vi "transRec.vi"() -> ()   [LabVIEW 2015]
uses:
  <vilib>/imath/engines/lvmath/Functions/Error Handling/error.ctl
  <instrlib>/niUSRP/niUSRP Write Tx Data (2D CDB).vi
  <instrlib>/niUSRP/niUSRP Fetch Rx Data (CDB WDT).vi
  <vilib>/measure/maspectr.llb/FFT Power Spectrum for 1 Chan (CDB).vi
  <vilib>/imath/engines/lvmath2/RunTimeEngine/Managers/WorkSpace/UID Generator.vi
  <vilib>/imath/engines/lvmath2/RunTimeEngine/NonStaticBuiltInFunctions/Manual/NIMS_NS_load.vi
  <vilib>/imath/engines/lvmath/Plug In/Control Design/NonStaticBuiltInFunctions/NIMS_NS_repeatmx.vi
  <vilib>/imath/engines/lvmath2/RunTimeEngine/RunTimeType/NIMS_RunTimeType_From StrictType (excl LVString).vi
  <instcachedir>/0/NIMS_RunTimeType_From StrictType (excl LVString)_EB1C38A9BC5048DA9ABDA8F781E54D21.lvgen/NIMS_RunTimeType_From StrictType (excl LVString)_EB1C38A9BC5048DA9ABDA8F781E54D21_000.vi
  <vilib>/imath/engines/lvmath2/RunTimeEngine/Managers/SymbolTable/Write Variable.vi
  <vilib>/imath/engines/lvmath/Plug In/Control Design/RunTimeSymbolToken/NIMS_CD_RunTimeSymbolToken_ResolveSymbol.vi
  <instcachedir>/0/NIMS_CD_RunTimeSymbolToken_ResolveSymbol_2FAE1C21E82D46CA9B9EE006FDCE72DC.lvgen/NIMS_CD_RunTimeSymbolToken_ResolveSymbol_2FAE1C21E82D46CA9B9EE006FDCE72DC_000.vi
  <vilib>/imath/engines/lvmath2/RunTimeEngine/LocalVariableDefStatement/MC_LocalVariableDefStatement_Display.vi
  <vilib>/imath/engines/lvmath2/RunTimeEngine/RunTimeSymbolToken/NIMS_RunTimeSymbolToken_ReadVariable-1out.vi
  <instcachedir>/0/NIMS_CD_RunTimeSymbolToken_ResolveSymbol_2FAE1C21E82D46CA9B9EE006FDCE72DC.lvgen/NIMS_CD_RunTimeSymbolToken_ResolveSymbol_2FAE1C21E82D46CA9B9EE006FDCE72DC_001.vi
  <vilib>/imath/engines/lvmath/Functions/Error Handling/MergeErrorsWrapper.vi
  <vilib>/imath/engines/lvmath2/RunTimeEngine/ArithmeticOperatorToken/NIMS_NS_ArithmeticOperator_rightdiv.vi
  <vilib>/imath/engines/lvmath/Plug In/Control Design/ArithmeticOperatorToken/NIMS_CD_NS_ArithmeticOperator_multmx.vi
  <vilib>/imath/engines/lvmath2/RunTimeEngine/CommandStatement/NIMS_CommandStatement_MaskErr.vi
  <vilib>/imath/engines/lvmath2/RunTimeEngine/Managers/SymbolTable/Read Variable.vi
  <vilib>/imath/engines/lvmath2/RunTimeEngine/RunTimeType/NIMS_RunTimeType_Get Case Value.vi
  <vilib>/imathl/engines/lvmath/Functions/Error Handling/Create Error.vi
  <vilib>/imath/engines/lvmath2/RunTimeEngine/RunTimeType/NIMS_RunTimeType_To Numeric.vi
  <instcachedir>/0/NIMS_RunTimeType_To Numeric_B134FEC7BFC54ED5998F4CFD2EE98288.lvgen/NIMS_RunTimeType_To Numeric_B134FEC7BFC54ED5998F4CFD2EE98288_000.vi
  <vilib>/imath/engines/lvmath/Plug In/_Char/RunTimeType/NIMS_CH_RunTimeType_To Character 2D.vi
  <vilib>/imath/engines/lvmath/Plug In/_Char/NIMS_CH_Character 2D to U8 2D.vi
  <vilib>/imath/engines/lvmath2/RunTimeEngine/NodeEndStatement/MC_NodeEndStatement_Dispose.vi
  <vilib>/imath/engines/lvmath2/RunTimeEngine/NodeEndStatement/NIMS_NodeEndStatement_Output.vi
  <instcachedir>/0/NIMS_NodeEndStatement_Output_53EC0D466D134D7ABD903AC30B43404B.lvgen/NIMS_NodeEndStatement_Output_53EC0D466D134D7ABD903AC30B43404B_003.vi
  <vilib>/imath/engines/lvmath2/RunTimeEngine/ErrorHandling/NIMS_Finalize Error.vi
  <vilib>/imath/engines/lvmath2/RunTimeEngine/Managers/SymbolTable/NIMS_WorkSpace.lvlib
  <vilib>/measure/NI_MAPro.lvlib
panel:
  out "Baseband Power Spectrum":cluster{"f0":dbl, "df":dbl, "magnitude":dbl[]}(graph)
  out "Waveform Graph 2":dbl[][](graph)
  out "Waveform Graph":dbl[][](graph)
  in  "error in rx":errorcluster
  in  "device names rx":refnum<k15>
  in  "active antenna x2":string
  in  "active antenna x1":string
  out "coerced gain x2":dbl format="%#_6f"
  out "coerced carrier frequency x2":dbl=100000.0 format="%#_6p"
  out "coerced IQ rate x2":dbl=100000.0 format="%#_6p"
  in  "gain x2":dbl format="%#_6f"
  in  "IQ rate x2":dbl=100000.0 format="%#_6p"
  in  "carrier frequency x2":dbl=100000.0 format="%#_6p"
  in  "device names x2":refnum<k15>
  in  "error in 2":errorcluster
  in  "stop button x2":bool
  in  "number of samples":i64=100000
  in  "stop button rx":bool
  in  "active antenna rx":string
  out "coerced carrier frequency rx":dbl=100000.0 format="%#_6p"
  out "coerced gain rx":dbl format="%#_6f"
  out "coerced IQ rate rx":dbl=100000.0 format="%#_6p"
  in  "gain rx":dbl format="%#_6f"
  in  "carrier frequency rx":dbl=100000.0 format="%#_6p"
  in  "IQ rate rx":dbl=100000.0 format="%#_6p"
  in  "stop button x1":bool
  out "coerced gain x1":dbl format="%#_6f"
  out "coerced carrier frequency x1":dbl=100000.0 format="%#_6p"
  out "coerced IQ rate x1":dbl=100000.0 format="%#_6p"
  in  "gain x1":dbl format="%#_6f"
  in  "IQ rate x1":dbl=100000.0 format="%#_6p"
  in  "carrier frequency x1":dbl=100000.0 format="%#_6p"
  in  "device names x1":refnum<k15>
  in  "error in 1":errorcluster
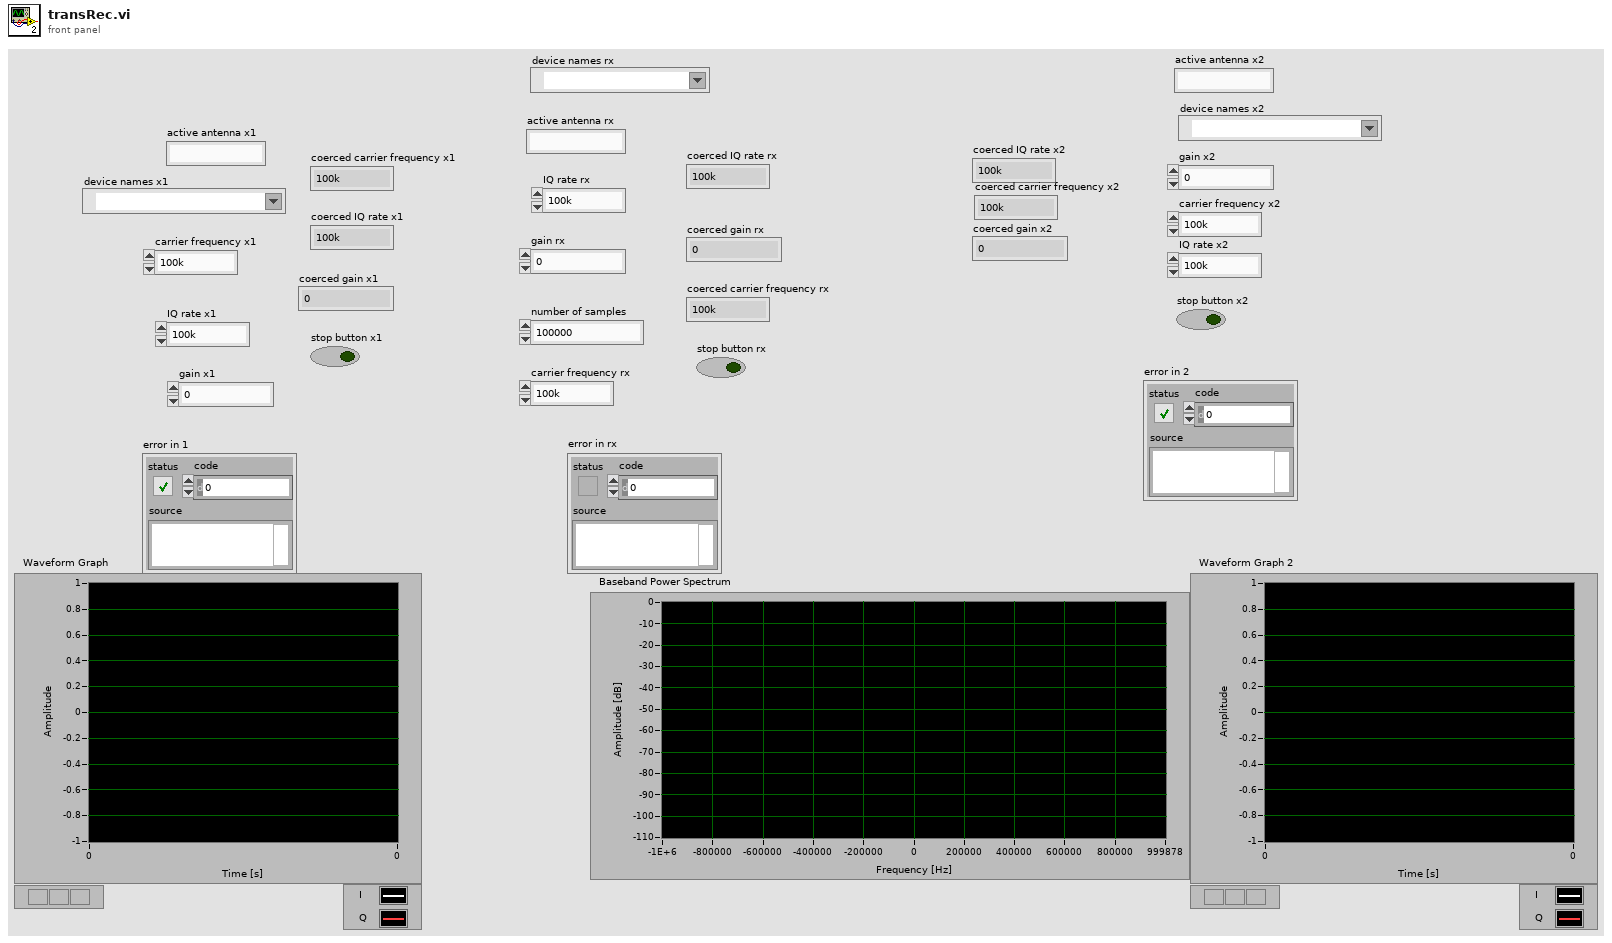
[diagram p1: front panel]
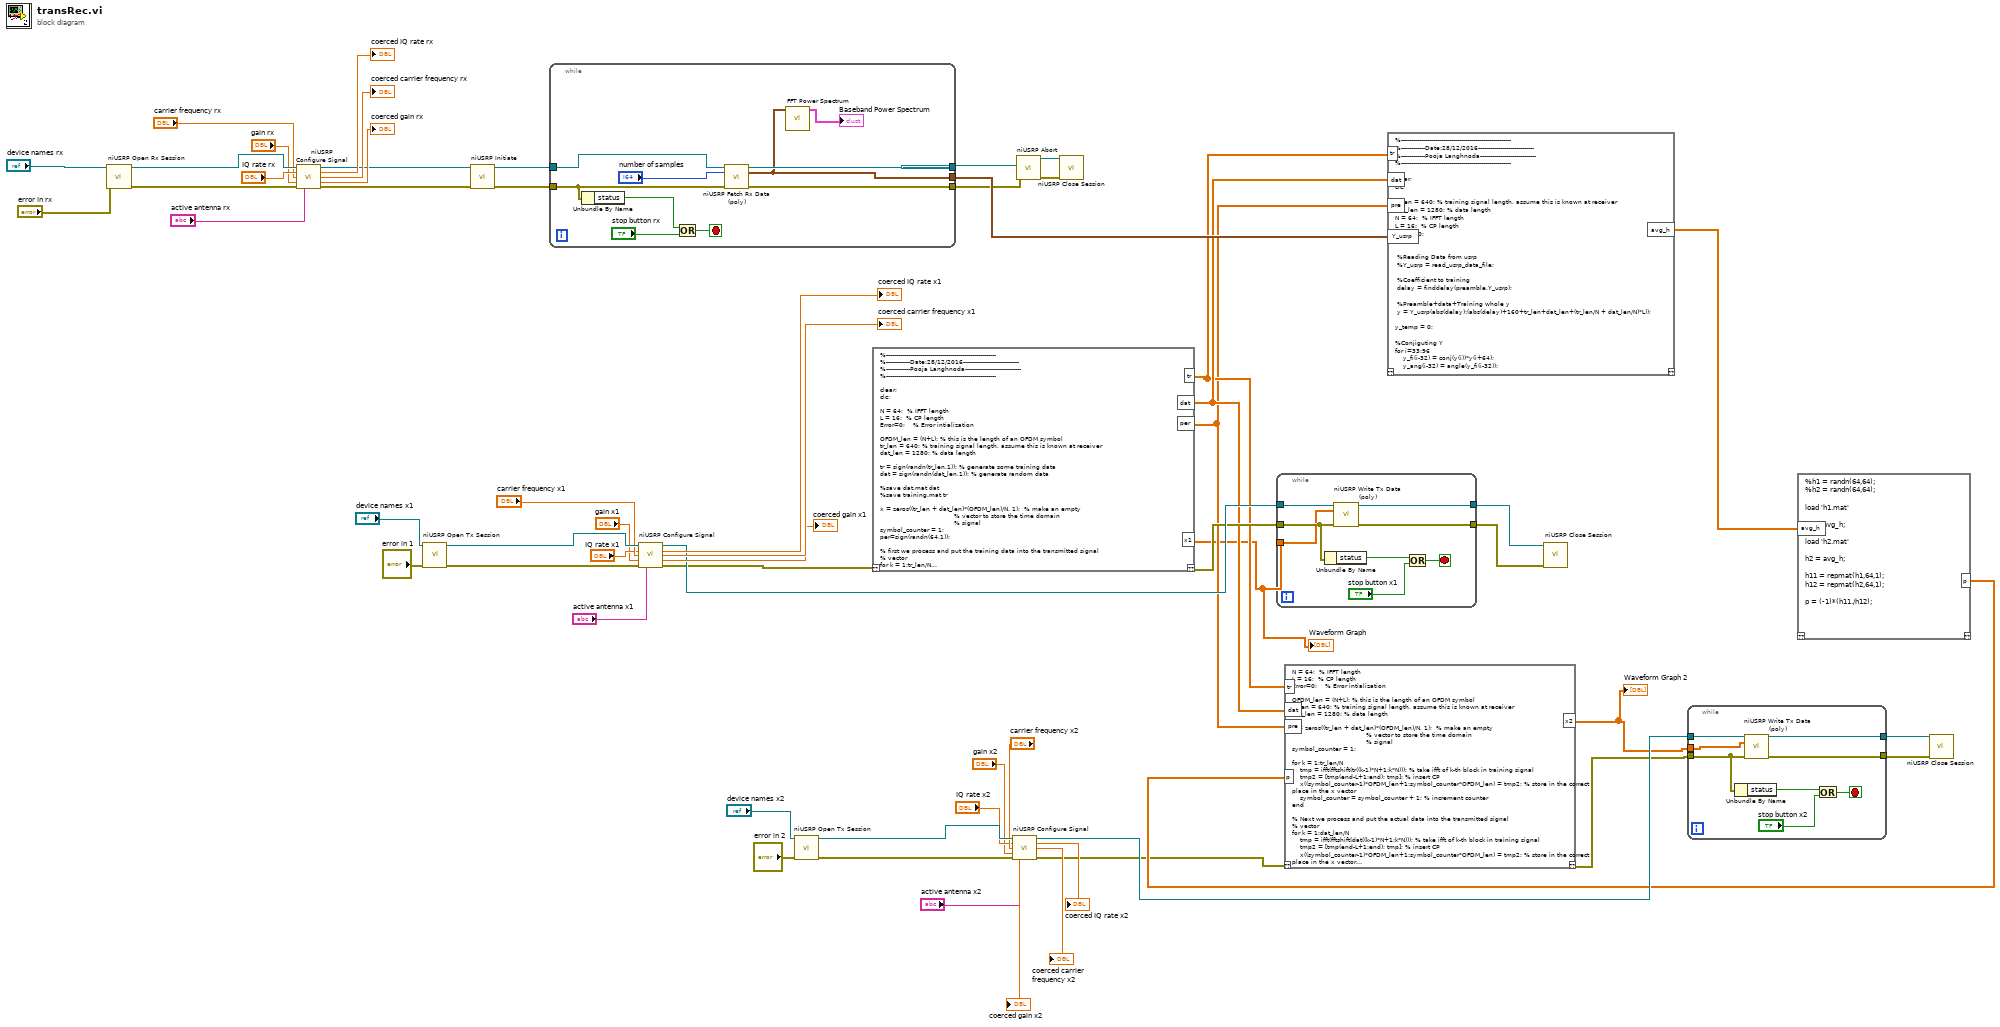
[diagram p0: block diagram]
diagram:
  n1 = call <instrlib>:"niUSRP Open Rx Session.vi"("device names"="device names rx", "error in (no error)"="error in rx") -> ("session handle out"=w45:refnum<k15>, "error out"=w44:errorcluster)  [unwired: 12 in]
  n2 = call <instrlib>:"niUSRP Configure Signal.vi"("session handle"=w45, "IQ rate"="IQ rate rx", "carrier frequency"="carrier frequency rx", "gain"="gain rx", "error in (no error)"=w44, "active antenna"="active antenna rx") -> ("session handle out"=w38:refnum<k15>, "coerced IQ rate"=→"coerced IQ rate rx":dbl, "coerced carrier frequency"=→"coerced carrier frequency rx":dbl, "coerced gain"=→"coerced gain rx":dbl, "error out"=w37:errorcluster)  [unwired: 5 in]
  n3 = call <instrlib>:"niUSRP Open Tx Session.vi"("device names"="device names x1", "error in (no error)"="error in 1") -> ("session handle out"=w58:refnum<k15>, "error out"=w50:errorcluster)  [unwired: 12 in]
  n4 = call <instrlib>:"niUSRP Initiate.vi"("session handle"=w38, "error in (no error)"=w37) -> ("session handle out"=w35:refnum<k15>, "error out"=w34:errorcluster)  [unwired: 12 in]
  n5 = while {
    tunnel: w35 -> [w65]
    tunnel: [w66] -> w30
    tunnel: w34 -> [w62]
    tunnel: [w61] -> w33
    tunnel: [w63] -> w29
    stop <- w67 stop-if-true
    n6 = Unbundle By Name(w62) -> ("status"=w68:bool)
    n7 = Or(x=w68, y="stop button rx") -> (x .or. y?=w67:bool)
    n8 = call-poly <instrlib>:"niUSRP Fetch Rx Data (poly).vi"("session handle"=w65, "number of samples"="number of samples", "error in (no error)"=w62) -> ("session handle out"=w66:refnum<k15>, "data"=w61:waveform(cdb), "error out"=w63:errorcluster)  [unwired: 9 in, 1 out]
    n9 = call-poly <vilib>:"FFT Power Spectrum.vi"("time signal"=w61) -> ("power spectrum"=→"Baseband Power Spectrum":cluster{"f0":dbl, "df":dbl, "magnitude":dbl[]})  [unwired: 7 in, 3 out]
  }
  n10 = call <instrlib>:"niUSRP Configure Signal.vi"("session handle"=w58, "IQ rate"="IQ rate x1", "carrier frequency"="carrier frequency x1", "gain"="gain x1", "error in (no error)"=w50, "active antenna"="active antenna x1") -> ("session handle out"=w49:refnum<k15>, "coerced IQ rate"=→"coerced IQ rate x1":dbl, "coerced carrier frequency"=→"coerced carrier frequency x1":dbl, "coerced gain"=→"coerced gain x1":dbl, "error out"=w8:errorcluster)  [unwired: 5 in]
  n11 = call <instrlib>:"niUSRP Open Tx Session.vi"("device names"="device names x2", "error in (no error)"="error in 2") -> ("session handle out"=w23:refnum<k15>, "error out"=w18:errorcluster)  [unwired: 12 in]
  n12 = script code="%-------------------------------------------------------\n%------------Date:28/12/2016----------------------------\n%------------Pooja Langhnoda----------------------------\n%-------------------------------------------------------\n\nclear;\nclc;\n\nN = 64;  % IFFT length\nL = 16;  % CP length\nError=0;    % Error intialization\n\nOFDM_len = (N+L); % this is the length of an OFDM symbol\ntr_len = 640; % training signal length, assume this is known at receiver\ndat_len = 1280; % data length\n\ntr = sign(randn(tr_len,1)); % generate some training data\ndat = sign(randn(dat_len,1)); % generate random data\n\n%save dat.mat dat\n%save training.mat tr\n\nx = zeros((tr_len + dat_len)*(OFDM_len)/N, 1);  % make an empty \n                                     % vector to store the time domain \n                                     % signal\nsymbol_counter = 1;\nper=sign(randn(64,1));\n\n% first we process and put the training data into the transmitted signal\n% vector\nfor k = 1:tr_len/N\n    tmp = ifft(fftshift(tr((k-1)*N+1:k*N))); % take ifft of k-th block in training signal\n    tmp2 = [tmp(end-L+1:end); tmp]; % insert CP\n    x((symbol_counter-1)*OFDM_len+1:symbol_counter*OFDM_len) = tmp2; % store in the correct place in the x vector\n    symbol_counter = symbol_counter + 1; % increment counter\nend\n\n% Next we process and put the actual data into the transmitted signal\n% vector\nfor k = 1:dat_len/N\n    tmp = ifft(fftshift(dat((k-1)*N+1:k*N))); % take ifft of k-th block in training signal\n    tmp2 = [tmp(end-L+1:end); tmp]; % insert CP\n    x((symbol_counter-1)*OFDM_len+1:symbol_counter*OFDM_len) = tmp2; % store in the correct place in the x vector\n    symbol_counter = symbol_counter + 1; % increment counter\nend\n\n% normalize signal to have unit power\nx=x./std(x);\n\n%concating preamble\nx= cat(1,per(33:64),per,per(1:64),x);\n\npre = x(1:160);\n%save preamble.mat pre\n\n%Writing data to USRP and file\n\n  x_usrp=x./10;\n  x1 = zeros(2*length(x_usrp),1);\n    x1(1:2:end) = real(x_usrp);\n    x1(2:2:end) = imag(x_usrp);"("??"=w8) -> ("??"=w46:errorcluster, "tr"=w27:dbl[][], "dat"=w28:dbl[][], "per"=w10:dbl[][], "x1"=w2:cdb[][])
  "Waveform Graph" <- w2
  n13 = call <instrlib>:"niUSRP Configure Signal.vi"("session handle"=w23, "IQ rate"="IQ rate x2", "carrier frequency"="carrier frequency x2", "gain"="gain x2", "error in (no error)"=w18, "active antenna"="active antenna x2") -> ("session handle out"=w17:refnum<k15>, "coerced IQ rate"=→"coerced IQ rate x2":dbl, "coerced carrier frequency"=→"coerced carrier frequency x2":dbl, "coerced gain"=→"coerced gain x2":dbl, "error out"=w5:errorcluster)  [unwired: 5 in]
  n14 = call <instrlib>:"niUSRP Abort.vi"("session handle"=w30, "error in (no error)"=w29) -> ("session handle out"=w32:refnum<k15>, "error out"=w31:errorcluster)  [unwired: 12 in]
  n15 = call <instrlib>:"niUSRP Close Session.vi"("session handle"=w32, "error in (no error)"=w31) -> ()  [unwired: 13 in, 1 out]
  n16 = while {
    tunnel: w49 -> [w71]
    tunnel: [w77] -> w48
    tunnel: w46 -> [w72]
    tunnel: [w73] -> w47
    tunnel: w2 -> [w70]
    stop <- w74 stop-if-true
    n17 = Unbundle By Name(w72) -> ("status"=w75:bool)
    n18 = call-poly <instrlib>:"niUSRP Write Tx Data (poly).vi"("session handle"=w71, "data"=w70, "error in (no error)"=w72) -> ("session handle out"=w77:refnum<k15>, "error out"=w73:errorcluster)  [unwired: 11 in]
    n19 = Or(x=w75, y="stop button x1") -> (x .or. y?=w74:bool)
  }
  n20 = script code="%-------------------------------------------------------\n%------------Date:28/12/2016----------------------------\n%------------Pooja Langhnoda----------------------------\n%-------------------------------------------------------\n\nclear;\nclc;\n\ntr_len = 640; % training signal length, assume this is known at receiver\ndat_len = 1280; % data length\nN = 64;  % IFFT length\nL = 16;  % CP length\nError = 0;\n \n \n %Reading Data from usrp\n %Y_usrp = read_usrp_data_file;\n \n %Coefficient to training\n delay = finddelay(preamble,Y_usrp);\n \n %Preamble+data+Training whole y\n y = Y_usrp(abs(delay):(abs(delay)+160+tr_len+dat_len+(tr_len/N + dat_len/N)*L));   \n \ny_temp = 0;\n\n%Conjiguting Y\nfor i=33:96\n    y_fi(i-32) = conj(y(i))*y(i+64);\n    y_ang(i-32) = angle(y_fi(i-32));\n\n    y_temp = y_temp + y_ang(i-32);\n    \nend\n\ny_avg = -y_temp/(64*64);\ndisplay(y_avg);\n\n%Removing exp()\nfor i=1:(length(y)-1)\n    y_rmv(i) = y(i)*(exp(1i*y_avg*i));\nend\n\n%Transposing the tr\nTr = transpose(tr);\nH_tmp = zeros(1,64);\n\n%Frequency Domain\nfor i=3:(tr_len/N+2)\n    \n    Y_tr((i-3)*64+1:(i-2)*64) = fftshift(fft(y_rmv((i-1)*80+17:i*80)));\n    \n    %Getting H Estimation\n    H = Y_tr((i-3)*64+1:(i-2)*64)./Tr((i-3)*64+1:(i-2)*64);\n    H_tmp = H_tmp + H;\nend\n\navg_h = H_tmp./10;\n%save h.mat avg_h\nplot(abs(avg_h));\n\nfor i=13:(dat_len/N+12)\n    %Taking FFT per block\n    y_data((i-13)*64+1:(i-12)*64) = fftshift(fft(y_rmv((i-1)*80+17:i*80)));  %freq domain\n  \n    %Getting x from Y and H\n    X((i-13)*64+1:(i-12)*64) = y_data((i-13)*64+1:(i-12)*64)./avg_h;\nend\n\nx_sign = sign(real(X));\n\n%checking Error\nfor k=1:dat_len\n    if((x_sign(k)>0 && dat(k)<0)||(x_sign(k)<0 && dat(k)>0))\n        Error = Error+1;\n    end\nend\n%Error bit\n   error = Error/dat_len;\n   display(error);"("tr"=w27, "pre"=w10, "dat"=w28, "Y_usrp"=w33) -> ("avg_h"=w15:cdb[][])  [unwired: 1 in, 1 out]
  n21 = call <instrlib>:"niUSRP Close Session.vi"("session handle"=w48, "error in (no error)"=w47) -> ()  [unwired: 13 in, 1 out]
  n22 = mathscript code="%h1 = randn(64,64);\n%h2 = randn(64,64);\n\nload 'h1.mat'\n\nh1 = avg_h;\n\nload 'h2.mat'\n\nh2 = avg_h;\n \nh11 = repmat(h1,64,1);\nh12 = repmat(h2,64,1);\n\np = (-1)*(h11./h12);"("avg_h"=w15) -> ("p"=w16:cdb[][])  [unwired: 1 in, 1 out]
  n23 = script code="N = 64;  % IFFT length\nL = 16;  % CP length\nError=0;    % Error intialization\n\nOFDM_len = (N+L); % this is the length of an OFDM symbol\ntr_len = 640; % training signal length, assume this is known at receiver\ndat_len = 1280; % data length\n\nx = zeros((tr_len + dat_len)*(OFDM_len)/N, 1);  % make an empty \n                                     % vector to store the time domain \n                                     % signal\nsymbol_counter = 1;\n\nfor k = 1:tr_len/N\n    tmp = ifft(fftshift(tr((k-1)*N+1:k*N))); % take ifft of k-th block in training signal\n    tmp2 = [tmp(end-L+1:end); tmp]; % insert CP\n    x((symbol_counter-1)*OFDM_len+1:symbol_counter*OFDM_len) = tmp2; % store in the correct place in the x vector\n    symbol_counter = symbol_counter + 1; % increment counter\nend\n\n% Next we process and put the actual data into the transmitted signal\n% vector\nfor k = 1:dat_len/N\n    tmp = ifft(fftshift(dat((k-1)*N+1:k*N))); % take ifft of k-th block in training signal\n    tmp2 = [tmp(end-L+1:end); tmp]; % insert CP\n    x((symbol_counter-1)*OFDM_len+1:symbol_counter*OFDM_len) = tmp2; % store in the correct place in the x vector\n    symbol_counter = symbol_counter + 1; % increment counter\nend\n\n% normalize signal to have unit power\nx=x./std(x);\n%concating preamble\nx= cat(1,per(33:64),per,per(1:64),x);\n\npreamble = x(1:160);\nx_temp=p.*x;\n\nx2 = zeros(2*length(x_temp),1);\n    x2(1:2:end) = real(x_temp);\n    x2(2:2:end) = imag(x_temp);"("??"=w5, "tr"=w27, "dat"=w28, "pre"=w10, "p"=w16) -> ("??"=w14:errorcluster, "x2"=w1:dbl[][])
  "Waveform Graph 2" <- w1
  n24 = while {
    tunnel: w17 -> [w79]
    tunnel: [w85] -> w26
    tunnel: w14 -> [w80]
    tunnel: [w81] -> w25
    tunnel: w1 -> [w78]
    stop <- w82 stop-if-true
    n25 = Unbundle By Name(w80) -> ("status"=w83:bool)
    n26 = call-poly <instrlib>:"niUSRP Write Tx Data (poly).vi"("session handle"=w79, "data"=w78, "error in (no error)"=w80) -> ("session handle out"=w85:refnum<k15>, "error out"=w81:errorcluster)  [unwired: 11 in]
    n27 = Or(x=w83, y="stop button x2") -> (x .or. y?=w82:bool)
  }
  n28 = call <instrlib>:"niUSRP Close Session.vi"("session handle"=w26, "error in (no error)"=w25) -> ()  [unwired: 13 in, 1 out]
